vi "Clear Measurement.vi"(8 "error in (no error)":errorcluster, 11 "VISA resource name":refnum<visa-resource-name>) -> (0 "error out":errorcluster, 3 "VISA resource name out":refnum<visa-resource-name>)   [LabVIEW 2009, in "Agilent 8000 Series.lvlib"]
doc: "Clears the measurement results from display and disables all previously enabled measurements."
uses:
  Agilent 8000 Series.lvlib
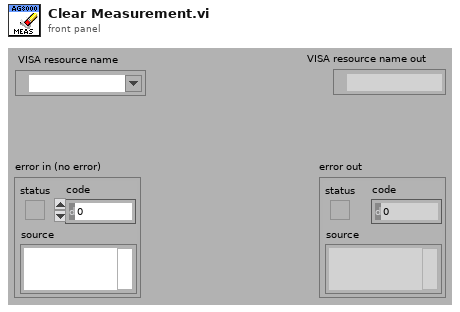
[diagram p1: front panel]
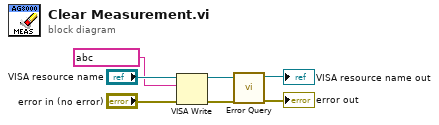
[diagram p0: block diagram]
diagram:
  n1 = VISA Write(VISA resource name="VISA resource name", write buffer=string ?, error in (no error)="error in (no error)") -> (VISA resource name out=w4:refnum<visa-resource-name>, error out=w3:errorcluster)  [unwired: 1 out]
  n2 = call "Error Query.vi"("error in (no error)"=w3, "VISA resource name"=w4) -> ("error out"=→"error out":errorcluster, "VISA resource name out"=→"VISA resource name out":refnum<visa-resource-name>)  [unwired: 6 in, 2 out]
